vi "Open 6.vi"(6 "Front Right Motor 2":T1=enum."Invalid", 7 "Rear Left Motor":T1=enum."Invalid", 8 "Front Right Motor 1":T1=enum."Invalid", 9 "Front Left Motor 2":T1=enum."Invalid", 10 "Front Left Motor 1":T1=enum."Invalid", 11 "Rear Right Motor":T1=enum."Invalid") -> (0 "error out":errorcluster, 3 "RobotDriveDevRef":T2={"DevStatus"={"status"=FALSE, "code"=0, "source"=""}, "Motors[]"=[], "Square Inputs"=FALSE, "Max Output"=1.0, "Isochronous"=FALSE})   [LabVIEW 2013]
uses:
  <vilib>/Rock Robotics/WPI/RobotDrive/WPI_RobotDriveDevRef.ctl
  <vilib>/Rock Robotics/WPI/MotorControl/WPI_MotorControlDeviceRef.ctl
  <vilib>/Rock Robotics/SystemInterfaces/Typedef/FPGA_TypedefDigitalModule.ctl
  <vilib>/Rock Robotics/SystemInterfaces/DIO/FPGA_DIOPWMChannel.ctl
  <vilib>/Rock Robotics/WPI/PWM/WPI_PWMDeadband.ctl
  <vilib>/Rock Robotics/WPI/CAN/Jaguar/SubVIs/WPI_CANJaguar_ControlMode.ctl
  <vilib>/Rock Robotics/WPI/PWM/WPI_PWMTransform_ConPane.ctl
  <vilib>/Rock Robotics/WPI/SafetyOutput/WPI_SafetyOutputConfigMenu.ctl
  <vilib>/Rock Robotics/WPI/MotorControl/WPI_MotorControlOpen Jaguar.vi
panel:
  in  "error in (no error)":errorcluster
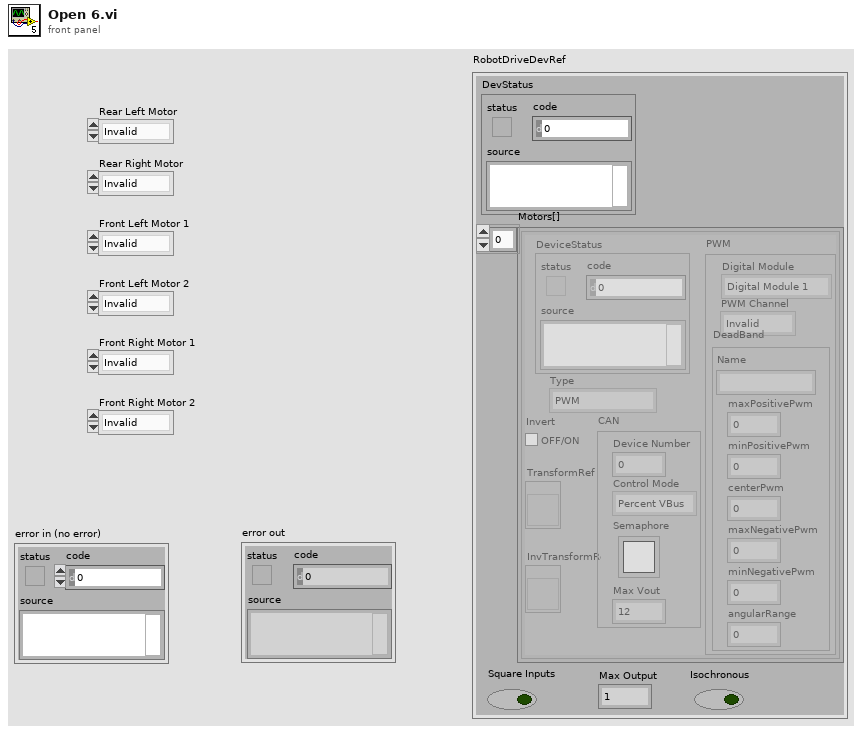
[diagram p1: front panel]
types:
  T1 = typedef "FPGA_DIOPWMChannel.ctl" = enum8{"PWM 1", "PWM 2", "PWM 3", "PWM 4", "PWM 5", "PWM 6", "PWM 7", "PWM 8", "PWM 9", "PWM 10", "Invalid"}
  T2 = typedef "WPI_RobotDriveDevRef.ctl" = cluster{"DevStatus":errorcluster, "Motors[]":T3[], "Square Inputs":bool, "Max Output":dbl, "Isochronous":bool}
  T3 = typedef "WPI_MotorControlDeviceRef.ctl" = cluster{"DeviceStatus":errorcluster, "Type":enum16{"PWM", "CAN"}, "PWM":cluster{"Digital Module":T4, "PWM Channel":T1, "DeadBand":T5}, "CAN":cluster{"Device Number":u8, "Control Mode":T6, "Semaphore":T7, "Max Vout":dbl}, "Invert":bool, "TransformRef":T8, "InvTransformRef":T8}
  T4 = typedef "FPGA_TypedefDigitalModule.ctl" = enum16{"Digital Module 1", "Digital Module 2"}
  T5 = typedef "WPI_PWMDeadband.ctl" = cluster{"Name":string, "maxPositivePwm":i32, "minPositivePwm":i32, "centerPwm":i32, "maxNegativePwm":i32, "minNegativePwm":i32, "angularRange":u16}
  T6 = typedef "WPI_CANJaguar_ControlMode.ctl" = enum8{"Percent VBus", "Current", "Speed", "Position", "Voltage"}
  T7 = typedef "Semaphore RefNum" = refnum<k1>
  T8 = typedef "WPI_PWMTransform_ConPane.ctl" = refnum<vi>
  T9 = typedef "WPI_SafetyOutputConfigMenu.ctl" = enum16{"Enable", "Disable"}
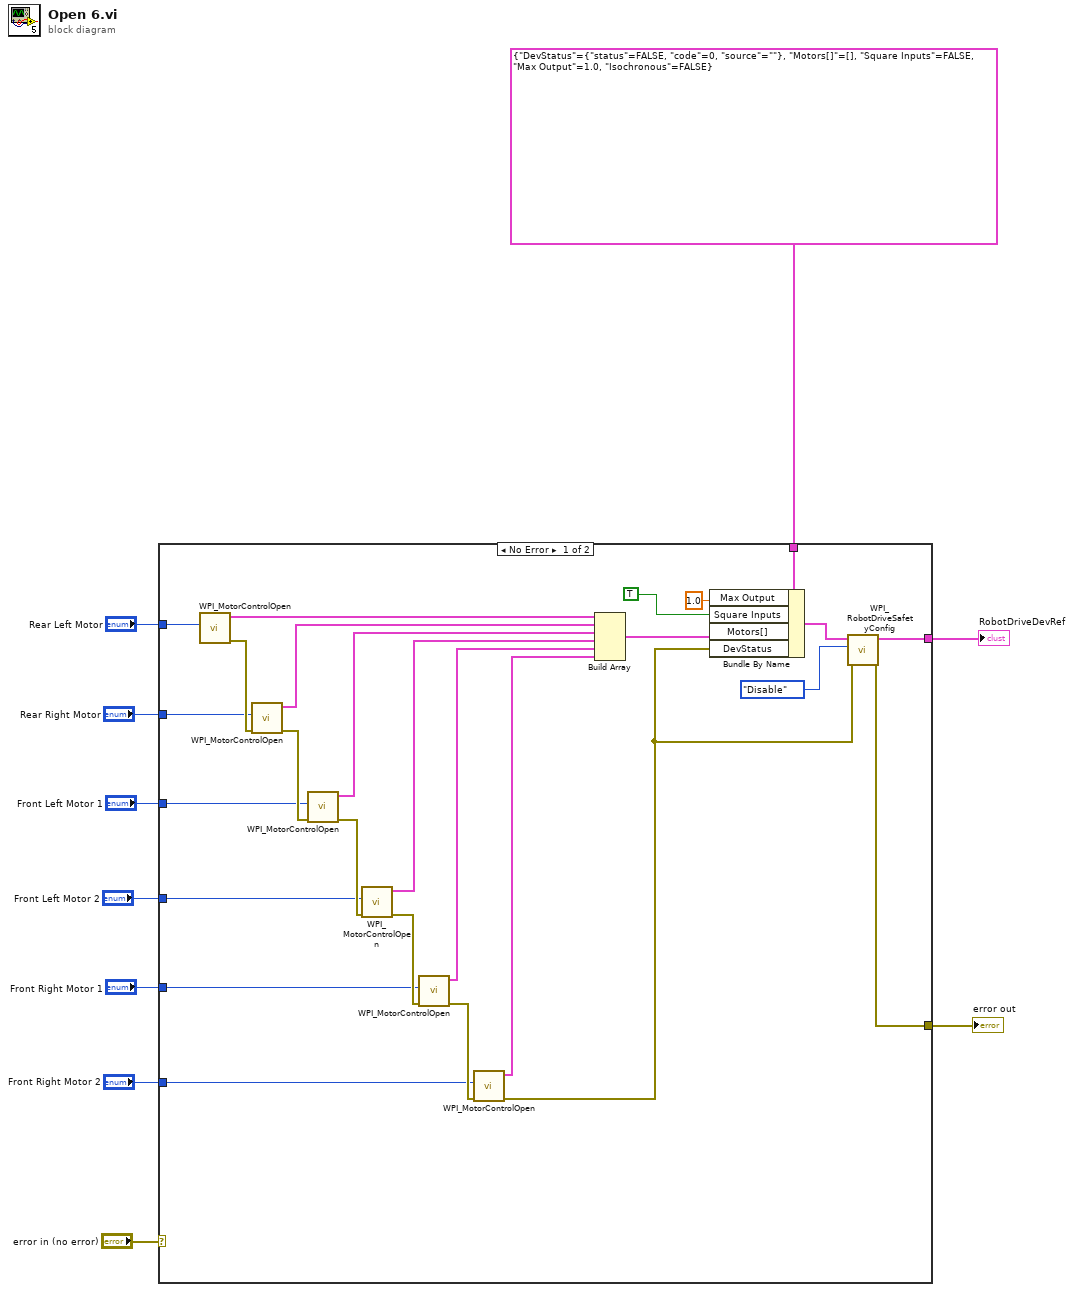
[diagram p0: block diagram]
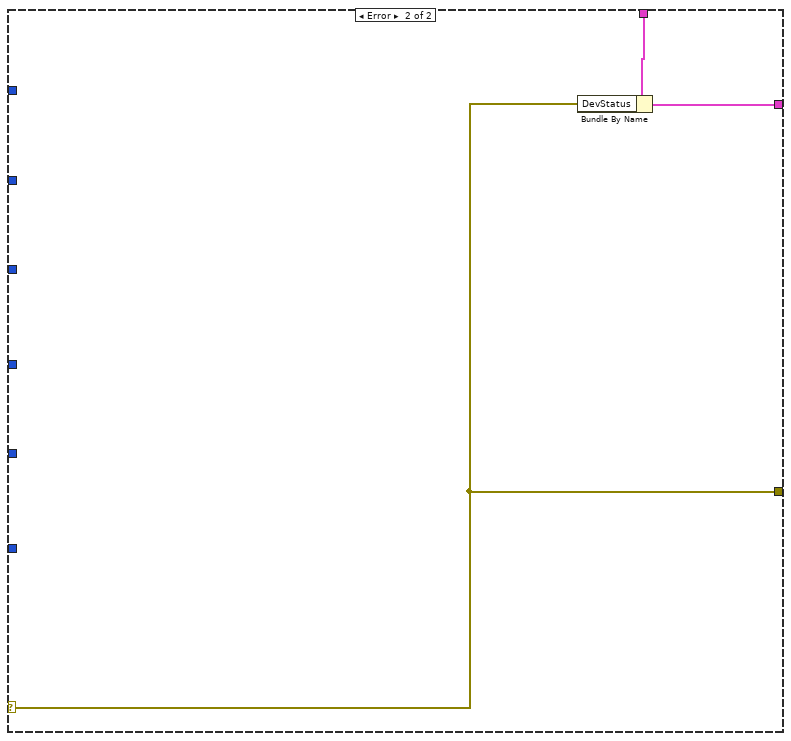
[diagram p2: hidden frame]
diagram:
  n1 = case shown="No Error" "error in (no error)" {
    selector: "error in (no error)" -> [_ w37]
    tunnel: [w23 w38] -> w7
    tunnel: T2 {"DevStatus"={"status"=FALSE, "code"=0, "source"=""}, "Motors[]"=[], "Square Inputs"=FALSE, "Max Output"=1.0, "Isochronous"=FALSE} ("RobotDriveDevRef") -> [w36 w39]
    tunnel: [w24 w37] -> w8
    tunnel: "Front Right Motor 2" -> [w16 _]
    tunnel: "Front Right Motor 1" -> [w15 _]
    tunnel: "Front Left Motor 2" -> [w14 _]
    tunnel: "Front Left Motor 1" -> [w13 _]
    tunnel: "Rear Right Motor" -> [w12 _]
    tunnel: "Rear Left Motor" -> [w11 _]
    frame No Error {
      n2 = call-poly <vilib>:"WPI_MotorControlOpen.vi"("PWM Channel"=w11) -> ("error out"=w28:errorcluster, "MotorControlDeviceRef"=w34:T3)  [unwired: 6 in, 3 out]
      n3 = call-poly <vilib>:"WPI_MotorControlOpen.vi"("error in (no error)"=w28, "PWM Channel"=w12) -> ("error out"=w29:errorcluster, "MotorControlDeviceRef"=w33:T3)  [unwired: 5 in, 3 out]
      n4 = call-poly <vilib>:"WPI_MotorControlOpen.vi"("error in (no error)"=w29, "PWM Channel"=w13) -> ("error out"=w30:errorcluster, "MotorControlDeviceRef"=w32:T3)  [unwired: 5 in, 3 out]
      n5 = call-poly <vilib>:"WPI_MotorControlOpen.vi"("error in (no error)"=w30, "PWM Channel"=w14) -> ("error out"=w20:errorcluster, "MotorControlDeviceRef"=w31:T3)  [unwired: 5 in, 3 out]
      n6 = call-poly <vilib>:"WPI_MotorControlOpen.vi"("error in (no error)"=w20, "PWM Channel"=w15) -> ("error out"=w21:errorcluster, "MotorControlDeviceRef"=w18:T3)  [unwired: 5 in, 3 out]
      n7 = call-poly <vilib>:"WPI_MotorControlOpen.vi"("error in (no error)"=w21, "PWM Channel"=w16) -> ("error out"=w19:errorcluster, "MotorControlDeviceRef"=w17:T3)  [unwired: 5 in, 3 out]
      n8 = Build Array(w34, w33, w32, w31, w18, w17) -> (w27:T3[])
      n9 = Bundle By Name(cluster=w36, "Max Output"=1.0, "Square Inputs"=TRUE ("DestroyPWM?"), "Motors[]"=w27, "DevStatus"=w19) -> (w25:T2)
      n10 = call <vilib>:"WPI_RobotDriveSafetyConfig.vi"("error in (no error)"=w19, "mode"=WPI_SafetyOutputConfigMenu."Disable", "RobotDriveDevRef"=w25) -> ("error out"=w24:errorcluster, "RobotDriveDevRef"=w23:T2)  [unwired: 1 in, 6 out]
    }
    frame Error {
      n11 = Bundle By Name(cluster=w39, "DevStatus"=w37) -> (w38:T2)
    }
  }
  "RobotDriveDevRef" <- w7
  "error out" <- w8
